vi "linear interpolation.vi"(7 "n":i32=-1, 11 "Array":cdb[](array[numeric])) -> (0 "interpolated average":cdb, 1 "mean":cdb, 2 "sum n z_n":cdb, 3 "sum z_n":cdb, 4 "slope":cdb, 6 "intercept":cdb)   [LabVIEW 2015]
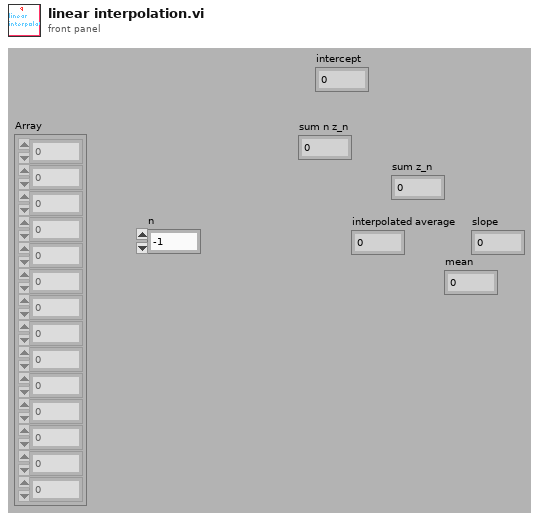
[diagram p1: front panel]
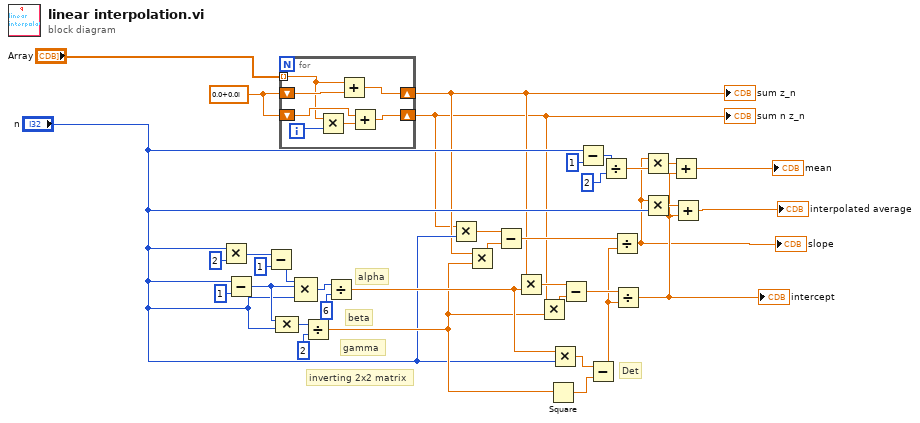
[diagram p0: block diagram]
diagram:
  w36 = cdb 0.0+0.0i
  # "inverting 2x2 matrix"
  # "Det"
  # "beta"
  # "gamma"
  # "alpha"
  n1 = Multiply(x="n", y=2 ("n")) -> (x*y=w32:i32)
  n2 = Subtract(x="n", y=1 ("n")) -> (x-y=w28:i32)
  n3 = Subtract(x=w32, y=1 ("n")) -> (x-y=w31:i32)
  n4 = Compound Arithmetic op=MULTIPLY(w28, "n") -> (w26:i32)
  n5 = for {
    tunnel: "Array" -> [w37] mode=indexing
    shift-right: [w43] -> w2
    shift-left: w36 -> [w42]
    shift-right: [w40] -> w1
    shift-left: w36 -> [w38]
    i -> [w39]
    n6 = Multiply(x=w37, y=w39) -> (x*y=w41:cdb)
    n7 = Add(x=w37, y=w42) -> (x+y=w43:cdb)
    n8 = Add(x=w38, y=w41) -> (x+y=w40:cdb)
  }
  "sum n z_n" <- w1
  "sum z_n" <- w2
  n9 = Compound Arithmetic op=MULTIPLY(w31, w28, "n") -> (w30:i32)
  n10 = Divide(x=w26, y=2 ("n")) -> (x/y=w17:dbl)
  n11 = Divide(x=w30, y=6 ("n")) -> (x/y=w18:dbl)
  n12 = Multiply(x=w1, y="n") -> (x*y=w22:cdb)
  n13 = Multiply(x=w2, y=w17) -> (x*y=w23:cdb)
  n14 = Subtract(x=w22, y=w23) -> (x-y=w21:cdb)
  n15 = Multiply(x=w2, y=w18) -> (x*y=w19:cdb)
  n16 = Multiply(x=w1, y=w17) -> (x*y=w20:cdb)
  n17 = Square(x=w17) -> (x^2=w24:dbl)
  n18 = Multiply(x=w18, y="n") -> (x*y=w25:dbl)
  n19 = Subtract(x=w19, y=w20) -> (x-y=w16:cdb)
  n20 = Subtract(x="n", y=1 ("n")) -> (x-y=w13:i32)
  n21 = Subtract(x=w25, y=w24) -> (x-y=w15:dbl)
  n22 = Divide(x=w13, y=2 ("n")) -> (x/y=w11:dbl)
  n23 = Divide(x=w21, y=w15) -> (x/y=w5:cdb)
  "slope" <- w5
  n24 = Divide(x=w16, y=w15) -> (x/y=w6:cdb)
  "intercept" <- w6
  n25 = Multiply(x=w5, y=w11) -> (x*y=w10:cdb)
  n26 = Multiply(x=w5, y="n") -> (x*y=w9:cdb)
  n27 = Add(x=w10, y=w6) -> (x+y=→"mean":cdb)
  n28 = Add(x=w9, y=w6) -> (x+y=→"interpolated average":cdb)
